vi "CSTK_MCListbox_Designer_UpdateColHdrsAttr.vi"(7 "表头属性列表输入":refnum<vi>, 8 "错误输入（无错误）":errorcluster, 11 "MCListbox引用句柄":refnum<vi>) -> (0 "错误输出":errorcluster, 2 "Selected Index":i32)   [LabVIEW 2015, in "CSTK_MCListbox Designer.lvlib"]
uses:
  CSTK_MCListbox Designer.lvlib
  _CSTK_MCListbox_Designer_ColHdr_Selected.ctl
  _CSTK_MCListbox_Designer_ColHdr.ctl
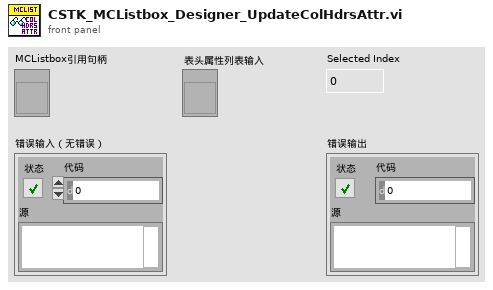
[diagram p1: front panel]
types:
  T1 = typedef "CSTK_MCListbox Designer.lvlib/_CSTK_MCListbox_Designer_ColHdr_Selected.ctl" = cluster{"选择":bool, "表头属性":T2}
  T2 = typedef "CSTK_MCListbox Designer.lvlib/_CSTK_MCListbox_Designer_ColHdr.ctl" = cluster{"列名称":string, "单元格宽度":u32, "粗体":bool, "斜体":bool, "对齐":enum16{"Left", "Center", "Right"}}
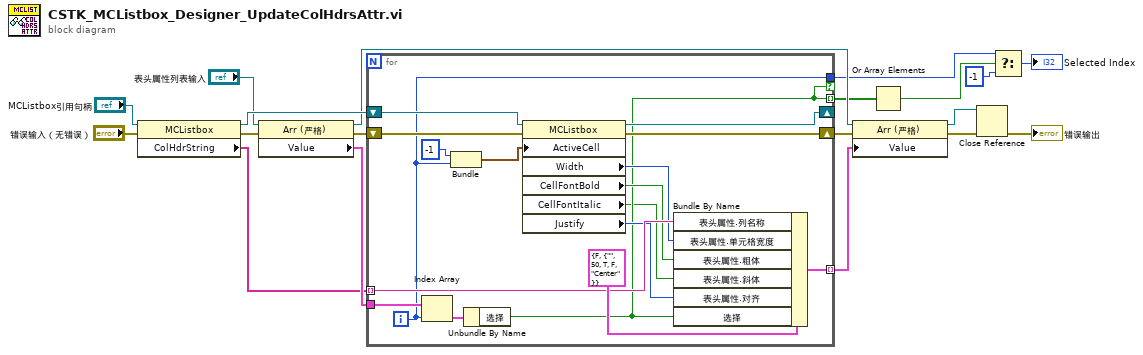
[diagram p0: block diagram]
diagram:
  n1 = property class="MCListbox"(reference="MCListbox引用句柄", error in="错误输入（无错误）") -> (reference out=w14:refnum<vi>, error out=w17:errorcluster, "ColHdrString"=w13:string[])
  n2 = property on="属性节点" class="Arr (严格)"(reference="表头属性列表输入", error in=w17) -> (reference out=w10:refnum<vi>, error out=w18:errorcluster, "Value"=w19:T1[])
  n3 = for {
    tunnel: w13 -> [w32] mode=indexing
    tunnel: [w28] -> w11 mode=indexing
    shift-right: [w25] -> w12
    shift-left: w18 -> [w26]
    shift-right: [w27] -> _
    shift-left: w14 -> [w36]
    tunnel: w19 -> [w24]
    tunnel: [w22] -> w4 if=w21
    tunnel: [w21] -> w6 mode=indexing
    i -> [w22]
    n4 = Index Array(array=w24, index=w22) -> (element=w23:T1)
    n5 = Bundle(-1, w22) -> (w34:cluster{i32, i32})  [unwired: 1 in]
    n6 = Unbundle By Name(w23) -> ("选择"=w21:bool)
    n7 = property class="MCListbox"(reference=w36, error in=w26, "ActiveCell"=w34) -> (reference out=w27:refnum<vi>, error out=w25:errorcluster, "Width"=w31:u32, "CellFontBold"=w30:bool, "CellFontItalic"=w20:bool, "Justify"=w29:enum16{"Left", "Center", "Right"})
    n8 = Bundle By Name(cluster=T1 {"选择"=FALSE, "表头属性"={"列名称"="", "单元格宽度"=50, "粗体"=TRUE, "斜体"=FALSE, "对齐"=enum."Center"}} ("表头属性"), "表头属性.列名称"=w32, "表头属性.单元格宽度"=w31, "表头属性.粗体"=w30, "表头属性.斜体"=w20, "表头属性.对齐"=w29, "选择"=w21) -> (w28:T1)
  }
  n9 = property on="属性节点" class="Arr (严格)"(reference=w10, error in=w12, "Value"=w11) -> (reference out=w9:refnum<vi>, error out=w8:errorcluster)
  n10 = Or Array Elements(Boolean array=w6) -> (logical OR=w5:bool)
  n11 = Close Reference(reference=w9, error in (no error)=w8) -> (error out=→"错误输出":errorcluster)
  n12 = Select(t=w4, s=w5, f=-1) -> (s? t:f=→"Selected Index":i32)
